vi "Text File Handler.vi"() -> ()   [LabVIEW 2013]
panel:
  out "data":string
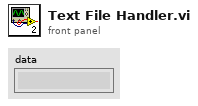
[diagram p1: front panel]
types:
  T1 = enum16{"создать", "добавить в начало", "добавить в конец", "считать", "очистить", "удалить", "пустий", ""}
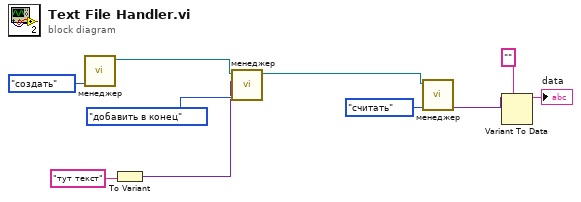
[diagram p0: block diagram]
diagram:
  n1 = call "менеджер.vi"("task"=T1."создать") -> ("queue out"=w8:refnum<queue>)  [unwired: 9 in, 1 out]
  n2 = To Variant(anything="тут текст") -> (Variant=w7:variant)
  n3 = call "менеджер.vi"("task"=T1."добавить в конец", "дані"=w7, "queue"=w8) -> ("queue out"=w4:refnum<queue>)  [unwired: 7 in, 1 out]
  n4 = call "менеджер.vi"("task"=T1."считать", "queue"=w4) -> ("дані вихід"=w3:variant)  [unwired: 8 in, 1 out]
  n5 = Variant To Data(type="", Variant=w3) -> (data=→"data":string)  [unwired: 1 in, 1 out]
